vi "Get Log Text Array From TDMS File.vi"(8 "error in":errorcluster, 10 "Group Name":string, 11 "Log File Path in":path) -> (0 "error out":errorcluster, 2 "Log Text Array":string[](array[string]), 3 "Log File Path out":path)   [LabVIEW 2020, in "TDMS Sink.lvclass"]
uses:
  TMDS Sink/TDMS Sink.lvclass
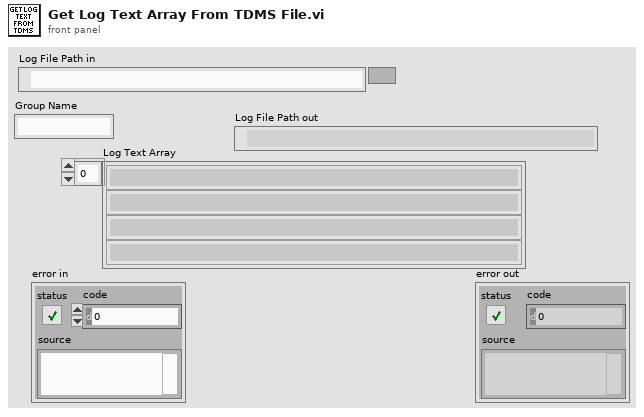
[diagram p1: front panel]
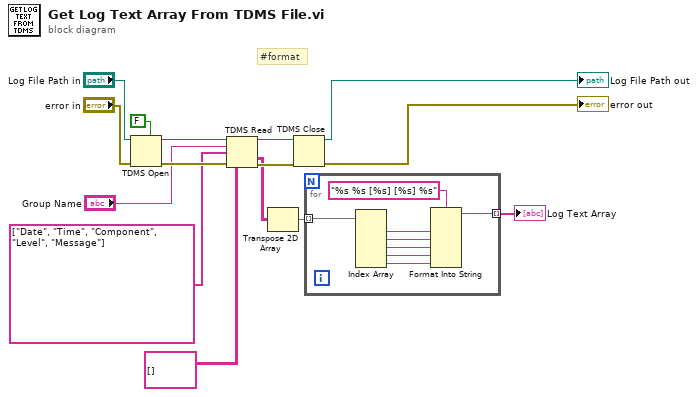
[diagram p0: block diagram]
diagram:
  # "#format"
  n1 = TDMS Open(5:FALSE ("create index file? (T)"), 8:"error in", 11:"Log File Path in") -> (0:w11:errorcluster, 3:w12:refnum<k34>)  [unwired: 4 in]
  n2 = TDMS Read(0:w12, 5:"Group Name", 7:string[] ["Date", "Time", "Component", "Level", "Message"] ("channel name(s) in (Untitled)"), 11:w11, 12:string[][] []) -> (4:w8:refnum<k34>, 10:w2:string[][], 15:w7:errorcluster)  [unwired: 3 in, 3 out]
  n3 = Transpose 2D Array(2D array=w2) -> (transposed array=w3:string[][])
  n4 = TDMS Close(8:w7, 11:w8) -> (0:→"error out":errorcluster, 3:→"Log File Path out":path)
  n5 = for {
    tunnel: w3 -> [w23] mode=indexing
    tunnel: [w16] -> w1 mode=indexing
    n6 = Index Array(array=w23) -> (element #1=w17:string, element #2=w18:string, element #3=w19:string, element #4=w20:string, element #5=w21:string)  [unwired: 5 in]
    n7 = Format Into String(format string="%s %s [%s] [%s] %s", w17, w18, w19, w20, w21) -> (resulting string=w16:string)  [unwired: 2 in, 1 out]
  }
  "Log Text Array" <- w1
